vi "Read Configure Current.vi"(11 "Digtal Multimeter in":refnum<class "Digital Multimeter.lvclass">) -> (2 "Configure Current":dbl, 3 "Digtal Multimeter out":refnum<class "Digital Multimeter.lvclass">)   [LabVIEW 2020, in "Digital Multimeter.lvclass"]
uses:
  Digital Multimeter.lvclass
  Digital Multimeter.lvclass/Digital Multimeter.ctl
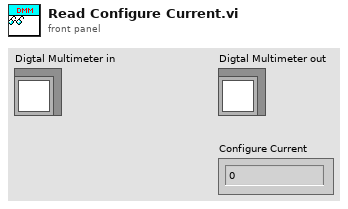
[diagram p1: front panel]
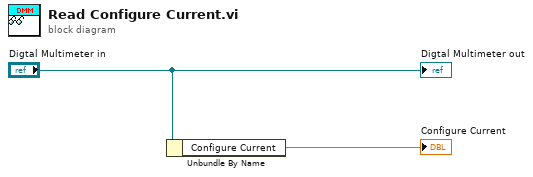
[diagram p0: block diagram]
diagram:
  n1 = Unbundle By Name("Digtal Multimeter in") -> ("Configure Current"=→"Configure Current":dbl)
  "Digtal Multimeter out" <- "Digtal Multimeter in"
